vi "Init Check.vi"(6 "Peripherals in":T1) -> (0 "error out":errorcluster, 1 "AISAS motors ok?":bool[](array[boolean]), 2 "auto off resp":string, 4 "Peripherals out":T1)   [LabVIEW 2014, in "AISAS Mech.lvclass"]
uses:
  AISAS Mech.lvclass
  Controls/peripherals.ctl
  AISAS Mech.lvclass/AISAS Mech.ctl
  Controls/Globals.vi
  Controls/Global demo.vi
  motor/AISAS motor.lvclass
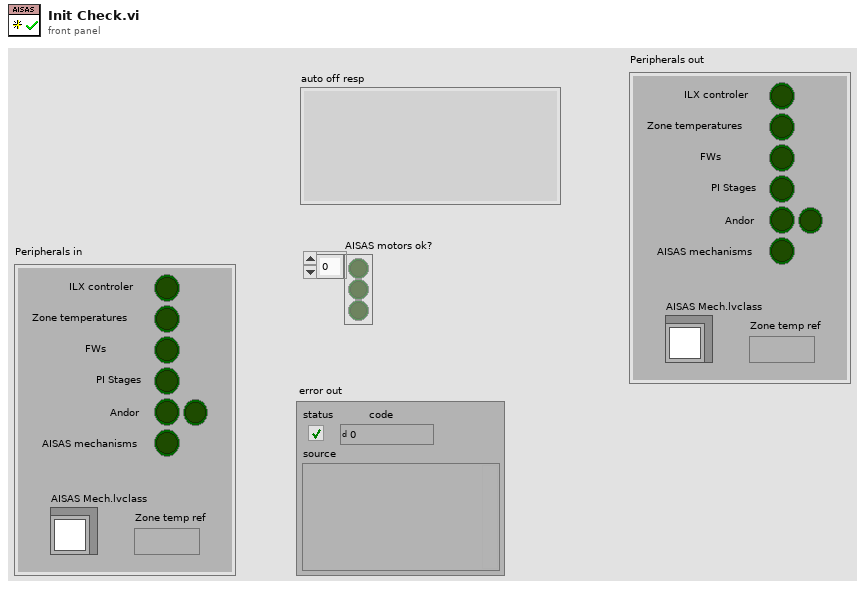
[diagram p1: front panel]
types:
  T1 = typedef "peripherals.ctl" = cluster{"ILX controler":bool, "Zone temperatures":bool, "Andor":bool, "Andor 2":bool, "PI Stages":bool, "AISAS mechanisms":bool, "AISAS Mech.lvclass":refnum<class "AISAS Mech.lvclass">, "Zone temp ref":variant, "FWs":bool}
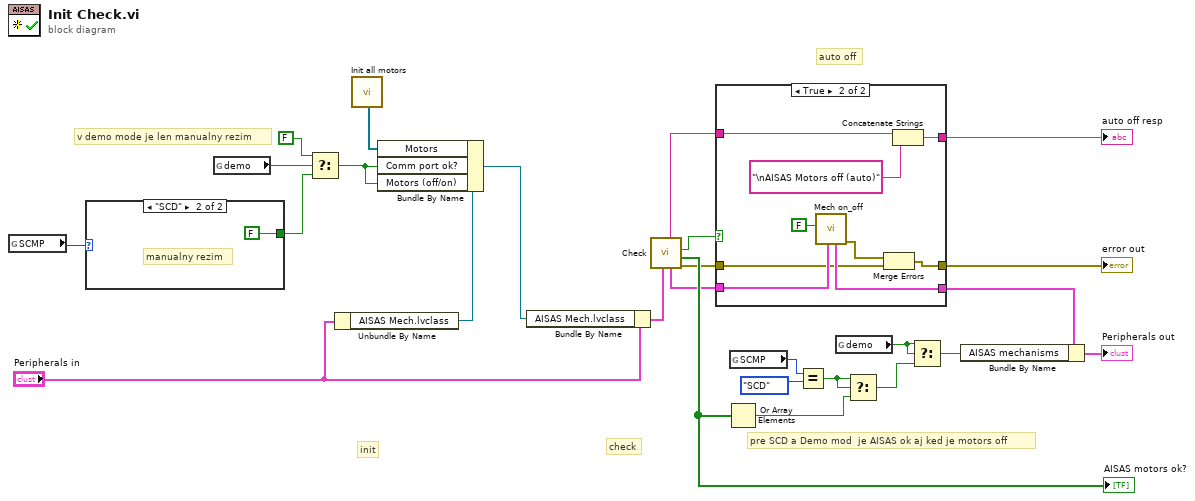
[diagram p0: block diagram]
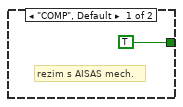
[diagram p3: hidden frame]
diagram:
  # "v demo mode je len manualny rezim"
  # "pre SCD a Demo mod  je AISAS ok aj ked je motors off"
  # "auto off"
  # "check"
  # "init"
  n1 = global read "Globals.vi" "SCMP"() -> (w25:enum16{"COMP", "SCD"})
  n2 = case shown="\"SCD\"" w25 {
    tunnel: [TRUE ("Motors (off/on)") FALSE ("Motors (off/on)")] -> w6
    frame "COMP", Default {
      # "rezim s AISAS mech."
    }
    frame "SCD" {
      # "manualny rezim"
    }
  }
  n3 = global read "Global demo.vi" "demo"() -> (w7:bool)
  n4 = Select(t=FALSE, s=w7, f=w6) -> (s? t:f=w5:bool)
  n5 = Unbundle By Name("Peripherals in") -> ("AISAS Mech.lvclass"=w24:refnum<class "AISAS Mech.lvclass">)
  n6 = call "Init all motors.vi"() -> ("AISAS Motors"=w26:refnum<class "AISAS motor.lvclass">[])  [unwired: 11 in]
  n7 = Bundle By Name(cluster=w24, "Motors"=w26, "Comm port ok?"=w5, "Motors (off/on)"=w5) -> (w22:refnum<class "AISAS Mech.lvclass">)
  n8 = Bundle By Name(cluster="Peripherals in", "AISAS Mech.lvclass"=w22) -> (w21:T1)
  n9 = call "Check.vi"("Peripherals in"=w21) -> ("error out"=w16:errorcluster, "motor ok?"=w19:bool[], "auto off?"=w18:bool, "Peripherals out"=w17:T1, "auto off resp"=w13:string)  [unwired: 6 in]
  "AISAS motors ok?" <- w19
  n10 = case shown="True" w18 {
    tunnel: w17 -> [w31 w40]
    tunnel: w16 -> [w30 w35]
    tunnel: [w31 w39] -> w15
    tunnel: [w30 w34] -> w14
    tunnel: w13 -> [w29 w32]
    tunnel: [w29 w36] -> w12
    frame False {
    }
    frame True {
      n11 = call "Mech on_off.vi"("Peripherals in"=w40, "Motors"=FALSE) -> ("error out"=w38:errorcluster, "Peripherals out"=w39:T1)  [unwired: 7 in, 1 out]
      n12 = Merge Errors(w38, w35) -> (w34:errorcluster)
      n13 = Concatenate Strings(w32, "\nAISAS Motors off (auto)" ("string")) -> (w36:string)
    }
  }
  "error out" <- w14
  "auto off resp" <- w12
  n14 = Or Array Elements(Boolean array=w19) -> (logical OR=w8:bool)
  n15 = global read "Globals.vi" "SCMP"() -> (w11:enum16{"COMP", "SCD"})
  n16 = Equal?(x=w11, y=enum16{"COMP", "SCD"}."SCD") -> (x = y?=w9:bool)
  n17 = global read "Global demo.vi" "demo"() -> (w1:bool)
  n18 = Select(t=w9, s=w9, f=w8) -> (s? t:f=w3:bool)
  n19 = Select(t=w1, s=w1, f=w3) -> (s? t:f=w2:bool)
  n20 = Bundle By Name(cluster=w15, "AISAS mechanisms"=w2) -> (→"Peripherals out":T1)
